vi "DHTxx Test Read Temperature.vi"() -> ()   [LabVIEW 2014, in "ESP8266 WiFi Wrapper.lvlib"]
uses:
  <vilib>/Aledyne-TSXperts/Arduino Compatible Compiler for LabVIEW/addons/ESP8266 WiFi Wrapper/ESP8266 WiFi Wrapper.lvlib
panel:
  out "Temperature":dbl
  out "Error Out":errorcluster
  in  "Error In":errorcluster
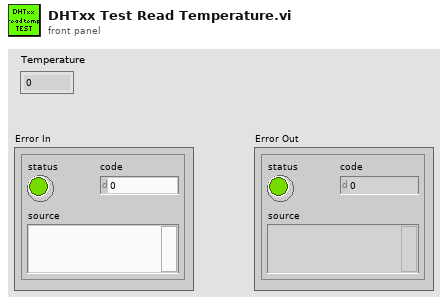
[diagram p1: front panel]
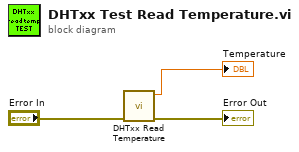
[diagram p0: block diagram]
diagram:
  n1 = call <vilib>:"DHTxx Read Temperature.vi"("Error In"="Error In") -> ("Error Out"=→"Error Out":errorcluster, "Temperature"=→"Temperature":dbl)  [unwired: 9 in]
